vi "MakeControlCode.vi"() -> (3 "resulting string":string="define hotloop(while (1) {if (#3C > 40.0) {relays&=11} if (#3C < 40.0){relays|=4} pause 0.1 s })")   [LabVIEW 2023]
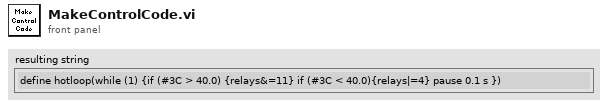
[diagram p1: front panel]
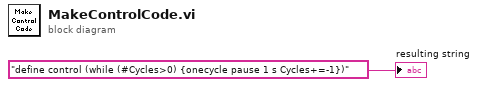
[diagram p0: block diagram]
diagram:
  "resulting string" <- "define control (while (#Cycles>0) {onecycle pause 1 s Cycles+=-1})" ("format string")
